vi "Imprimante sélection.vi"(2 "entrée d'erreur":errorcluster, 3 "Choix imprimante":T1(ring)) -> (0 "sortie d'erreur":errorcluster, 1 "Output ressource VISA":refnum<visa-resource-name>="none")   [LabVIEW 2020]
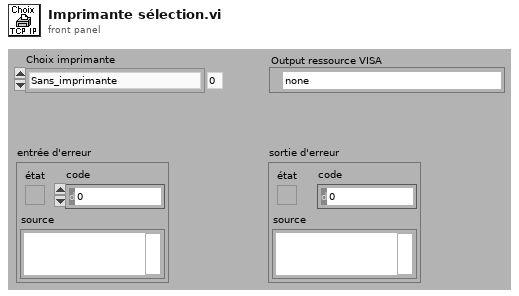
[diagram p1: front panel]
types:
  T1 = enum16{"Sans_imprimante", "Zebra_Medic_emballage2", "Zebra_Medic_2", "Zebra_Medic_1", "Zebra_Flat_emballage"}
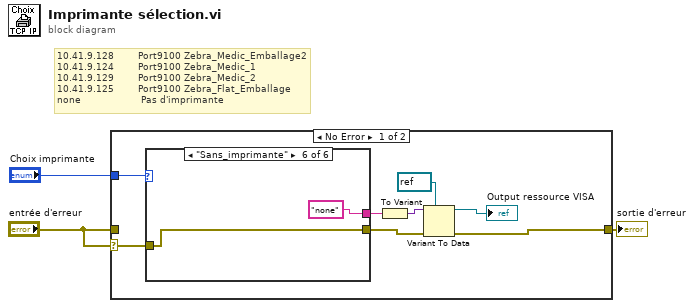
[diagram p0: block diagram]
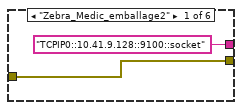
[diagram p2: hidden frame]
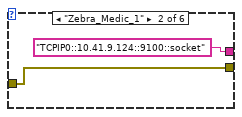
[diagram p3: hidden frame]
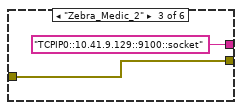
[diagram p4: hidden frame]
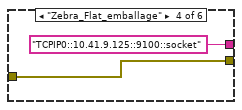
[diagram p5: hidden frame]
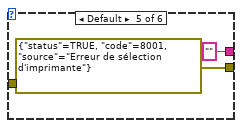
[diagram p6: hidden frame]
diagram:
  # "10.41.9.128\t       Port9100\tZebra_Medic_Emballage2\n10.41.9.124       \tPort9100\tZebra_Medic_1    \n10.41.9.129\t       Port9100\tZebra_Medic_2\n10.41.9.125       \tPort9100\tZebra_Flat_Emballage\nnone                    Pas d'imprimante"
  n1 = case shown="No Error" "entrée d'erreur" {
    selector: "entrée d'erreur" -> [w5 _]
    tunnel: [w7 w24] -> w3
    tunnel: "entrée d'erreur" -> [_ w24]
    tunnel: "Choix imprimante" -> [w6 _]
    frame No Error {
      n2 = case shown="\"Sans_imprimante\"" w6 {
        tunnel: ["TCPIP0::10.41.9.128::9100::socket" "TCPIP0::10.41.9.124::9100::socket" "TCPIP0::10.41.9.129::9100::socket" "TCPIP0::10.41.9.125::9100::socket" "" "none"] -> w11
        tunnel: w5 -> [w13 w15 w16 w19 _ w22]
        tunnel: [w13 w15 w16 w19 errorcluster {"status"=TRUE, "code"=8001, "source"="Erreur de sélection d'imprimante"} ("error IO") w22] -> w4
        frame "Zebra_Medic_emballage2" {
        }
        frame "Zebra_Medic_1" {
        }
        frame "Zebra_Medic_2" {
        }
        frame "Zebra_Flat_emballage" {
        }
        frame Default {
        }
        frame "Sans_imprimante" {
        }
      }
      n3 = To Variant(anything=w11) -> (Variant=w10:variant)
      n4 = Variant To Data(error in=w4, type=refnum<visa-resource-name> refnum ("Nom de ressource VISA en sortie"), Variant=w10) -> (data=→"Output ressource VISA":refnum<visa-resource-name>, error out=w7:errorcluster)
    }
    frame Error {
    }
  }
  "sortie d'erreur" <- w3
